vi "zero_pole_gain_to_filter.vi"(6 "Fs":dbl, 10 "Zero/Pole/Gain":cluster{" Zeros":T1[], "Poles":T1[], "Gain":dbl}={" Zeros"=[], "Poles"=[], "Gain"=1.0} {"Poles"."Frequency" format="%#_3p"; "Poles"."Damping" min=0.0 max=1000.0 step=1.0 format="%#_3g"; "Zeros"."Frequency" format="%#_3p"; "Zeros"."Damping" min=0.0 max=1000.0 step=1.0 format="%#_3g"}) -> (2 "IIR Filter Cluster":T2 {"Forward Coefficients" format="%#_4g"; "Reverse Coefficients" format="%#_4g"})   [LabVIEW 2010]
uses:
  damping_freq.ctl
panel:
  # "Create an arbitrary filter given specifications for the frequency and damping of the pole-zero pairs and desired DC gain (default 1).  Inverse of filter_to_zero_pole_gain.  This can be passed to any IIR filter VI."
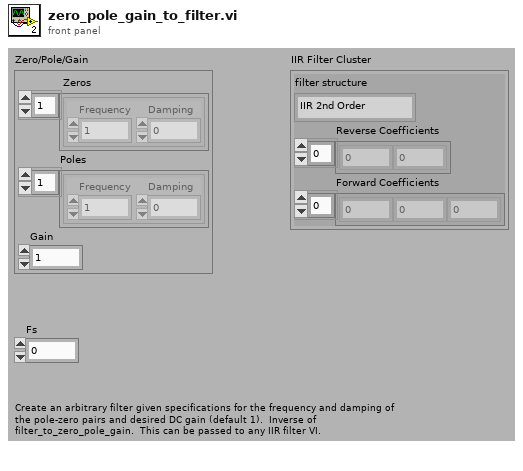
[diagram p1: front panel]
types:
  T1 = typedef "damping_freq.ctl" = cluster{"Frequency":dbl, "Damping":dbl}
  T2 = cluster{"filter structure":enum32{"IIR 2nd Order", "IIR 4th Order"}, "Reverse Coefficients":dbl[], "Forward Coefficients":dbl[]}
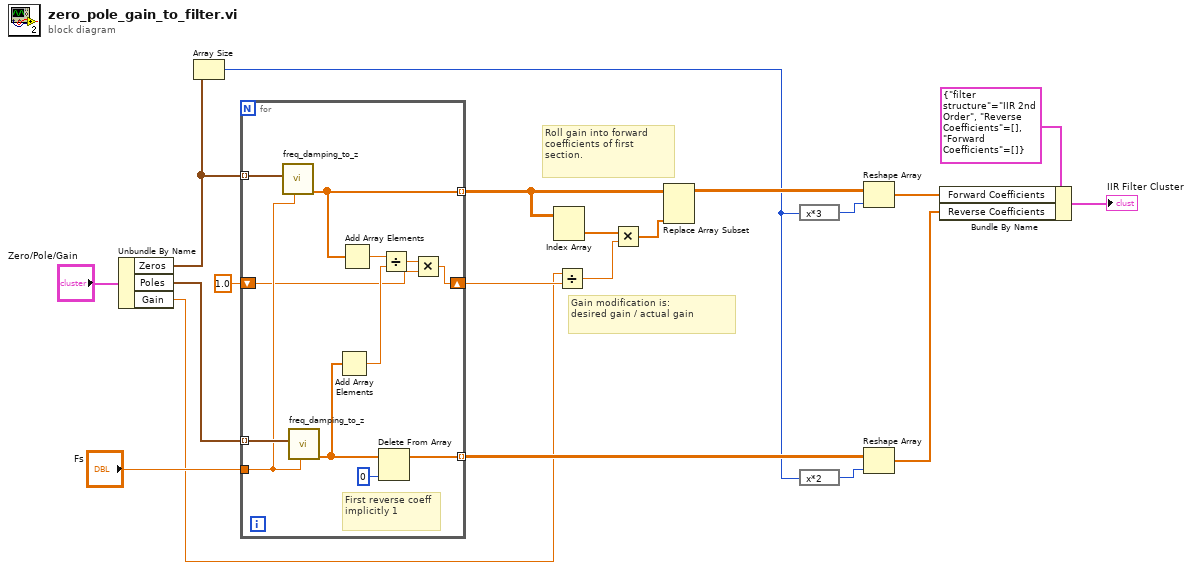
[diagram p0: block diagram]
diagram:
  # "Gain modification is:\ndesired gain / actual gain"
  # "Roll gain into forward coefficients of first section."
  n1 = Unbundle By Name("Zero/Pole/Gain") -> ("Zeros"=w6:T1[], "Poles"=w5:T1[], "Gain"=w2:dbl)
  n2 = Array Size(array=w6) -> (size(s)=w10:i32)
  n3 = for {
    tunnel: w5 -> [w32] mode=indexing
    tunnel: w6 -> [w31] mode=indexing
    tunnel: "Fs" -> [w30]
    tunnel: [w27] -> w14 mode=indexing
    tunnel: [w28] -> w11 mode=indexing
    shift-right: [w21] -> w3
    shift-left: 1.0 -> [w22]
    # "First reverse coeff implicitly 1"
    n4 = call "freq_damping_to_z.vi"("Fs"=w30, "Characteristics"=w31) -> ("Coefficients"=w27:dbl[])  [unwired: 9 out]
    n5 = call "freq_damping_to_z.vi"("Fs"=w30, "Characteristics"=w32) -> ("Coefficients"=w26:dbl[])  [unwired: 9 out]
    n6 = Add Array Elements(numeric array=w26) -> (sum=w24:dbl)
    n7 = Add Array Elements(numeric array=w27) -> (sum=w25:dbl)
    n8 = Delete From Array(array=w26, index=0) -> (array with subset deleted=w28:dbl[])  [unwired: 1 in, 1 out]
    n9 = Divide(x=w25, y=w24) -> (x/y=w23:dbl)
    n10 = Multiply(x=w23, y=w22) -> (x*y=w21:dbl)
  }
  n11 = Index Array(array=w14) -> (element=w15:dbl[])  [unwired: 2 in]
  n12 = Divide(x=w2, y=w3) -> (x/y=w1:dbl)
  n13 = Multiply(x=w15, y=w1) -> (x*y=w13:dbl[])
  n14 = Replace Array Subset(array=w14, new element=w13) -> (w12:dbl[][])  [unwired: 2 in]
  n15 = expression code="x*3"(w10) -> (w17:i32)
  n16 = expression code="x*2"(w10) -> (w16:i32)
  n17 = Reshape Array(w12, w17) -> (w9:dbl[])
  n18 = Reshape Array(w11, w16) -> (w8:dbl[])
  n19 = Bundle By Name(cluster=T2 {"filter structure"=enum."IIR 2nd Order", "Reverse Coefficients"=[], "Forward Coefficients"=[]} ("IIR Filter Cluster"), "Forward Coefficients"=w9, "Reverse Coefficients"=w8) -> (→"IIR Filter Cluster":T2)
